vi "Control PID - V1.vi"(5 "action":enum16{"CHECK", "INIT"}(ring), 6 "ITC temperature":dbl, 8 "error in":errorcluster, 11 "sweep folder path":path=path "E:/data/Ultrasound/Experiment/ProbeTest/Probe10/YBCO_6/sweep4") -> (0 "error out":errorcluster, 1 "PID":dbl[](array[numeric]), 2 "OK?":bool)   [LabVIEW 2014]
uses:
  ctl -- name dispatcher -- action.ctl
  itc 503 box - control.ctl
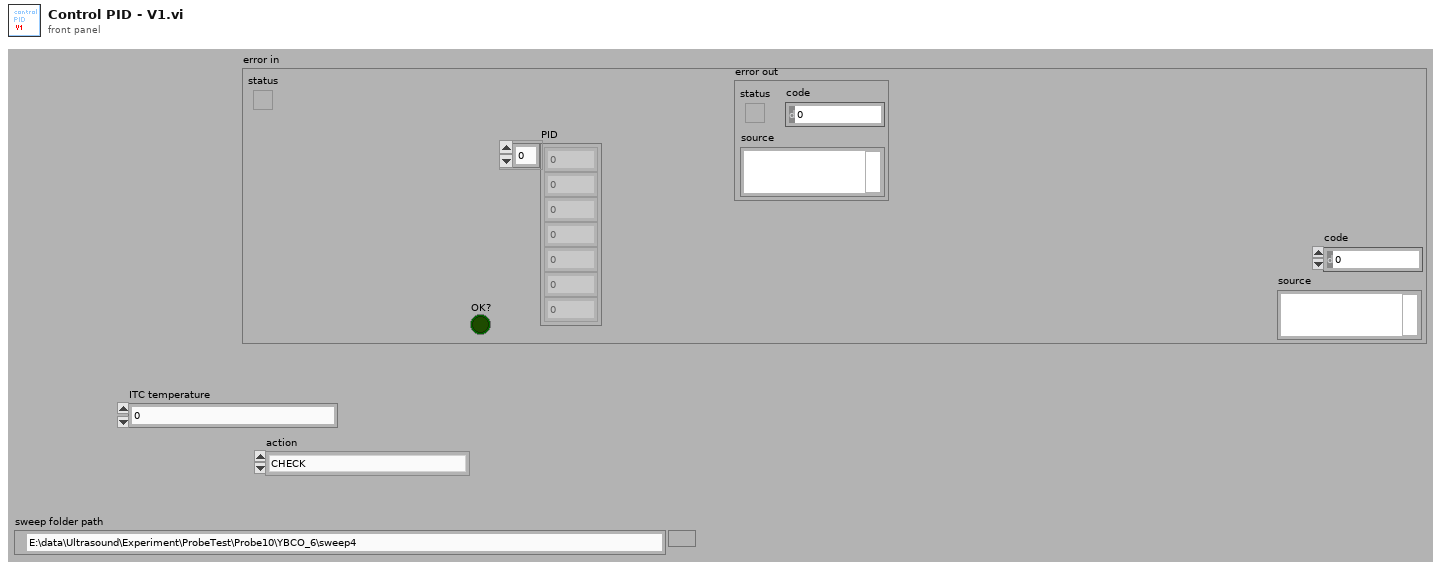
[diagram p1: front panel]
types:
  T1 = typedef "ctl -- name dispatcher -- action.ctl" = enum16{"peak frequency", "peak frequency DUMP", "peak gamma DUMP", "peak gamma", "peak frequency TEST", "peak gamma TEST", "ultrasonic power", "time in gamma", "set temperature ", "set temperature timer", "peak default gamma", "last scan file", "peak freq gamma TEST", "peak NAMES", "errors", "P_I_D", "P", "I", "D", "power vs time", "power vs time TIMER", "void", "power log", "set temperature - SINE", "itc ltc log", "peak - time in gamma"}
  T2 = typedef "itc 503 box - control.ctl" = enum16{"heater manual and zero", "heater auto", "upload D", "upload I", "upload P", "shut off", "init", "read sweep table", "disable", "enable", "read state", "set gas to", "stop sweep", "start sweep", "test", "set temperature to", "write sweep table", "-void", "set heater to"}
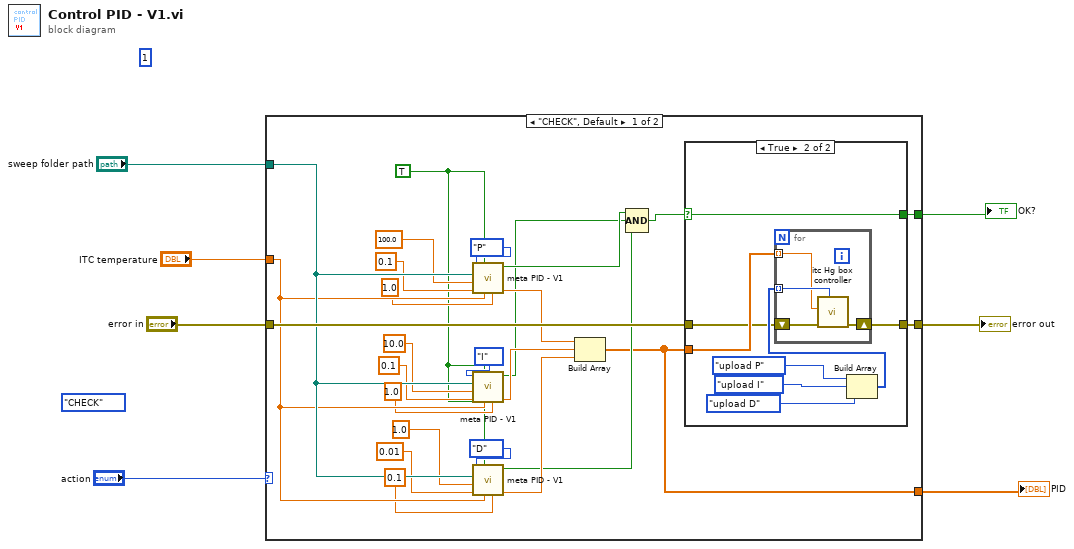
[diagram p0: block diagram]
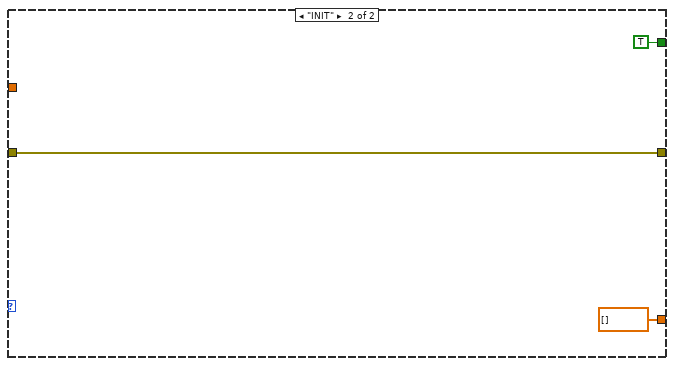
[diagram p3: hidden frame]
diagram:
  (unwired) enum16{"CHECK", "INIT"}."CHECK" ("action")
  (unwired) 1
  n1 = case shown="\"CHECK\", Default" "action" {
    tunnel: "ITC temperature" -> [w24 _]
    tunnel: "error in" -> [w33 w50]
    tunnel: [w32 w50] -> w5
    tunnel: "sweep folder path" -> [w25 _]
    tunnel: [w10 TRUE] -> w2
    tunnel: [w8 dbl[] []] -> w1
    frame "CHECK", Default {
      w9 = TRUE ("control power PID?")
      n2 = call "meta PID - V1.vi"("default output"=1.0 ("default"), "input parameter"=w24, "control?"=w9, "lower limit"=0.1 ("lower"), "upper limit"=100.0 ("upper"), "sweep folder path"=w25, "ctl name dispatch"=ctl_--_name_dispatcher_--_action."P") -> ("bezier output"=w30:dbl, "ok"=w23:bool)  [unwired: 1 in, 2 out]
      n3 = call "meta PID - V1.vi"("default output"=1.0 ("default"), "input parameter"=w24, "control?"=w9, "lower limit"=0.1 ("lower"), "upper limit"=10.0 ("upper"), "sweep folder path"=w25, "ctl name dispatch"=ctl_--_name_dispatcher_--_action."I") -> ("bezier output"=w28:dbl, "ok"=w22:bool)  [unwired: 1 in, 2 out]
      n4 = call "meta PID - V1.vi"("default output"=0.1 ("default"), "input parameter"=w24, "control?"=w9, "lower limit"=0.01 ("lower"), "upper limit"=1.0 ("upper"), "sweep folder path"=w25, "ctl name dispatch"=ctl_--_name_dispatcher_--_action."D") -> ("bezier output"=w29:dbl, "ok"=w21:bool)  [unwired: 1 in, 2 out]
      n5 = Build Array(w30, w28, w29) -> (w8:dbl[])
      n6 = Compound Arithmetic op=AND(w23, w22, w21) -> (w20:bool)
      n7 = case shown="True" w20 {
        selector: w20 -> [w34 w36]
        tunnel: w33 -> [w35 w37]
        tunnel: [w35 w43] -> w32
        tunnel: w8 -> [_ w38]
        tunnel: [w34 w36] -> w10
        frame False {
        }
        frame True {
          n8 = Build Array(itc_503_box_-_control."upload P" ("itc box action"), itc_503_box_-_control."upload I" ("itc box action"), itc_503_box_-_control."upload D" ("itc box action")) -> (w39:T2[])
          n9 = for {
            tunnel: w39 -> [w46] mode=indexing
            tunnel: w38 -> [w45] mode=indexing
            shift-right: [w47] -> w43
            shift-left: w37 -> [w44]
            n10 = call "itc Hg box controller.vi"("itc box action"=w46, "error in"=w44, "input"=w45) -> ("error out"=w47:errorcluster)  [unwired: 6 in, 2 out]
          }
        }
      }
    }
    frame "INIT" {
    }
  }
  "error out" <- w5
  "OK?" <- w2
  "PID" <- w1
